vi "Tree selection 1D search greater than.vi"(7 "Compare type":T1, 9 "Start index (0)":i32, 10 "Element":i32, 11 "1D array":i32[](array[numeric])) -> (3 "index of element":i32)   [LabVIEW 2020, in "UI_ItemSelect_OpenSource.lvlib"]
uses:
  UI_ItemSelect_OpenSource.lvlib
  tree item select search compare type.ctl
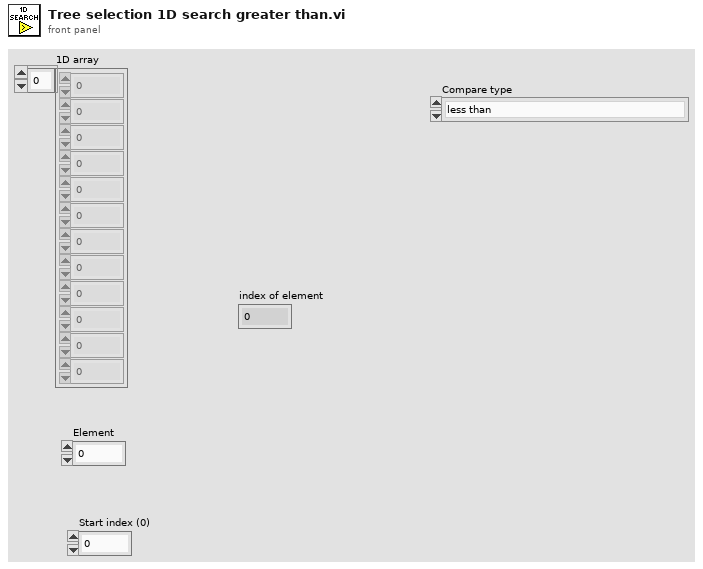
[diagram p1: front panel]
types:
  T1 = typedef "UI_ItemSelect_OpenSource.lvlib/tree item select search compare type.ctl" = enum16{"less than", "less than or equal", "greater than", "greater than or equal"}
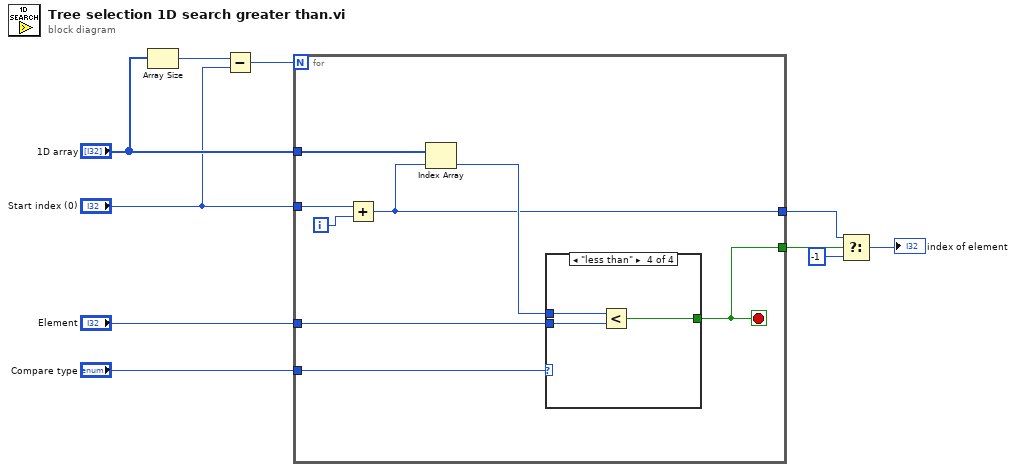
[diagram p0: block diagram]
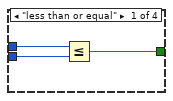
[diagram p2: hidden frame]
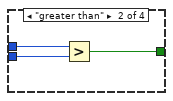
[diagram p3: hidden frame]
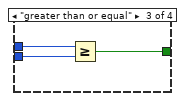
[diagram p4: hidden frame]
diagram:
  n1 = Array Size(array="1D array") -> (size(s)=w4:i32)
  n2 = Subtract(x=w4, y="Start index (0)") -> (x-y=w2:i32)
  n3 = for {
    N: w2 -> [_]
    tunnel: "1D array" -> [w18]
    tunnel: "Start index (0)" -> [w17]
    tunnel: "Element" -> [w15]
    tunnel: [w12] -> w8
    tunnel: [w13] -> w9
    tunnel: "Compare type" -> [w11]
    i -> [w16]
    stop <- w13 stop-if-true
    n4 = Add(x=w17, y=w16) -> (x+y=w12:i32)
    n5 = Index Array(array=w18, index=w12) -> (element=w14:i32)
    n6 = case shown="\"less than\"" w11 {
      tunnel: w15 -> [w21 w24 w27 w30]
      tunnel: w14 -> [w20 w23 w26 w29]
      tunnel: [w19 w22 w25 w28] -> w13
      frame "less than or equal" {
        n7 = Less Or Equal?(x=w20, y=w21) -> (x <= y?=w19:bool)
      }
      frame "greater than" {
        n8 = Greater?(x=w23, y=w24) -> (0:w22:bool)
      }
      frame "greater than or equal" {
        n9 = Greater Or Equal?(x=w26, y=w27) -> (x >= y?=w25:bool)
      }
      frame "less than" {
        n10 = Less?(x=w29, y=w30) -> (x < y?=w28:bool)
      }
    }
  }
  n11 = Select(t=w8, s=w9, f=-1) -> (s? t:f=→"index of element":i32)
